vi "GetCollision.vi"(4 "TheirSize":T2, 5 "MySize":T2, 6 "TheirPosition":T2, 7 "MyPosition":T2, 8 "error in (no error)":errorcluster, 11 "Velocity":T1) -> (0 "error out":errorcluster, 2 "direction_y":T3, 3 "direction_x":T3)   [LabVIEW 2019, in "RT_Game.lvlib" / "GameObject.lvclass"]
uses:
  GameObject/GameObject.lvclass
  Direction.ctl
  Game/Coordinate.ctl
  PongBall/Velocity.ctl
  RT_Game.lvlib
  Game/Game.lvclass
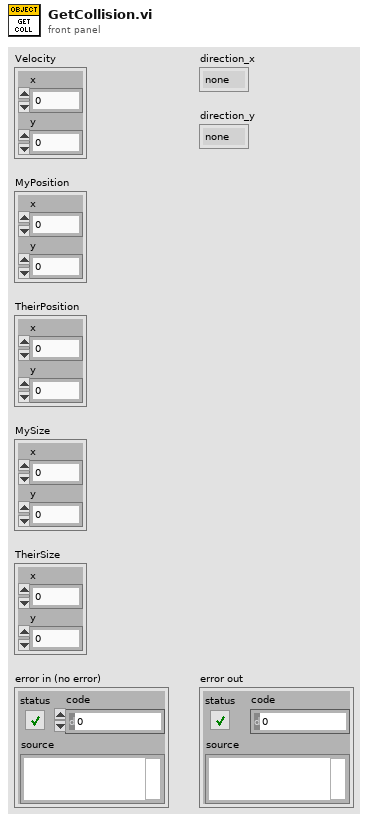
[diagram p1: front panel]
types:
  T1 = typedef "RT_Game.lvlib/Velocity.ctl" = cluster{"x":dbl, "y":dbl}
  T2 = typedef "RT_Game.lvlib/Game.lvclass/Coordinate.ctl" = cluster{"x":dbl, "y":dbl}
  T3 = typedef "RT_Game.lvlib/Direction.ctl" = enum16{"none", "Both", "left", "right", "up", "down"}
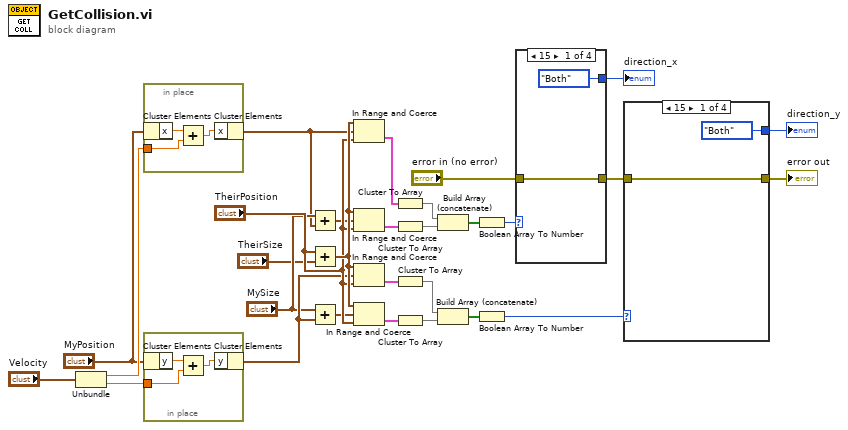
[diagram p0: block diagram]
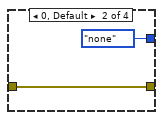
[diagram p2: hidden frame]
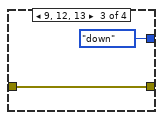
[diagram p3: hidden frame]
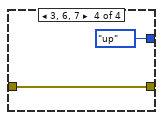
[diagram p4: hidden frame]
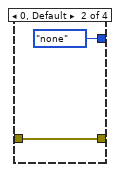
[diagram p5: hidden frame]
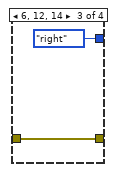
[diagram p6: hidden frame]
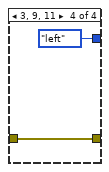
[diagram p7: hidden frame]
diagram:
  n1 = Unbundle("Velocity") -> ("x"=w3:dbl, "y"=w4:dbl)
  n2 = in-place {
    in-place-border: w3 -> [w31]
    n3 = in-place-cluster #1("MyPosition") -> ("x"=w32:dbl)
    n4 = Add(x=w32, y=w31) -> (x+y=w30:dbl)
    n5 = in-place-cluster #1("x"=w30) -> (w6:T2)
  }
  n6 = in-place {
    in-place-border: w4 -> [w34]
    n7 = in-place-cluster #2("MyPosition") -> ("y"=w35:dbl)
    n8 = Add(x=w35, y=w34) -> (x+y=w33:dbl)
    n9 = in-place-cluster #2("y"=w33) -> (w22:T2)
  }
  n10 = Add(x="MySize", y=w6) -> (x+y=w7:T2)
  n11 = Add(x="TheirPosition", y="TheirSize") -> (x+y=w24:T2)
  n12 = Add(x="MySize", y=w22) -> (x+y=w20:T2)
  n13 = In Range and Coerce(upper limit=w24, x=w6, lower limit="TheirPosition") -> (In Range?=w8:cluster{"x":bool, "y":bool})  [unwired: 1 out]
  n14 = In Range and Coerce(upper limit=w24, x=w7, lower limit="TheirPosition") -> (In Range?=w11:cluster{"x":bool, "y":bool})  [unwired: 1 out]
  n15 = In Range and Coerce(upper limit=w24, x=w22, lower limit="TheirPosition") -> (In Range?=w19:cluster{"x":bool, "y":bool})  [unwired: 1 out]
  n16 = In Range and Coerce(upper limit=w24, x=w20, lower limit="TheirPosition") -> (In Range?=w16:cluster{"x":bool, "y":bool})  [unwired: 1 out]
  n17 = Cluster To Array(cluster=w8) -> (array=w9:bool[])
  n18 = Cluster To Array(cluster=w11) -> (array=w12:bool[])
  n19 = Cluster To Array(cluster=w19) -> (array=w18:bool[])
  n20 = Cluster To Array(cluster=w16) -> (array=w15:bool[])
  n21 = Build Array (concatenate)(w9, w12) -> (w10:bool[])
  n22 = Build Array (concatenate)(w18, w15) -> (w17:bool[])
  n23 = Boolean Array To Number(Boolean array=w10) -> (number=w13:u32)
  n24 = Boolean Array To Number(Boolean array=w17) -> (number=w14:u32)
  n25 = case shown="15" w13 {
    tunnel: "error in (no error)" -> [w36 w39 w41 w43]
    tunnel: [w36 w39 w41 w43] -> w25
    tunnel: [Direction."Both" Direction."none" Direction."right" Direction."left"] -> w28
    frame 15 {
    }
    frame 0, Default {
    }
    frame 6, 12, 14 {
    }
    frame 3, 9, 11 {
    }
  }
  "direction_x" <- w28
  n26 = case shown="15" w14 {
    tunnel: [w45 w47 w49 w51] -> w27
    tunnel: w25 -> [w45 w47 w49 w51]
    tunnel: [Direction."Both" Direction."none" Direction."down" Direction."up"] -> w29
    frame 15 {
    }
    frame 0, Default {
    }
    frame 9, 12, 13 {
    }
    frame 3, 6, 7 {
    }
  }
  "direction_y" <- w29
  "error out" <- w27
